vi "Lossy Debug Enqueue.vi"(0 "Experimental Configuration":T1) -> ()   [LabVIEW 2013]
uses:
  Experimental Configuration.ctl
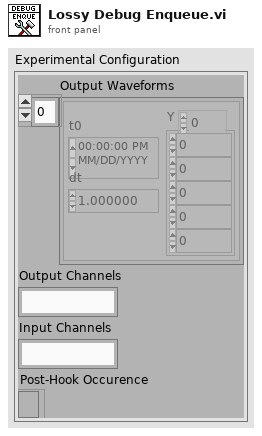
[diagram p1: front panel]
types:
  T1 = typedef "Experimental Configuration.ctl" = cluster{"Output Waveforms":waveform(dbl)[], "Output Channels":string, "Input Channels":string, "Post-Hook Occurence":refnum<k4>}
  T2 = typedef "Sidecar Debug Queue.ctl" = refnum<queue>
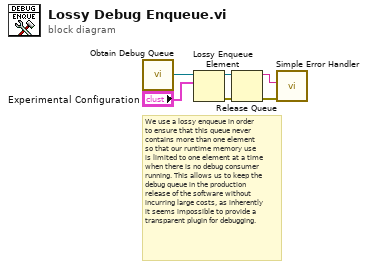
[diagram p0: block diagram]
diagram:
  # "We use a lossy enqueue in order\nto ensure that this queue never\ncontains more than one element\nso that our runtime memory use\nis limited to one element at a time\nwhen there is no debug consumer \nrunning. This allows us to keep the\ndebug queue in the production \nrelease of the software without \nincurring large costs, as inherently\nit seems impossible to provide a\ntransparent plugin for debugging."
  n1 = call "Obtain Debug Queue.vi"() -> ("Debug Queue"=w6:T2)
  n2 = Lossy Enqueue Element(queue=w6, element="Experimental Configuration") -> (queue out=w4:T2, error out=w3:errorcluster)  [unwired: 1 in, 2 out]
  n3 = Release Queue(queue=w4, error in (no error)=w3) -> (queue name=w1:string, error out=w2:errorcluster)  [unwired: 1 in, 1 out]
  n4 = call <vilib>:"Simple Error Handler.vi"("error source (\" \")"=w1, "error in (no error)"=w2) -> ()  [unwired: 3 in, 5 out]
